vi "GitCheckProcRepo.vi"(8 "error in (no error)":errorcluster, 9 "Directory":path=path "", 11 "Git exec":string="git") -> (0 "error out":errorcluster, 1 "Directory out":path, 2 "ProcedureRepo?":bool, 3 "Git exec out":string="git")   [LabVIEW 2013]
uses:
  GitInterface/GitCmd.vi
  <vilib>/dlg_ctls.llb/Space Constant.vi
  PathtoDirPath.vi
  <vilib>/Platform/system.llb/System Exec.vi
  <vilib>/Utility/error.llb/Error Cluster From Error Code.vi
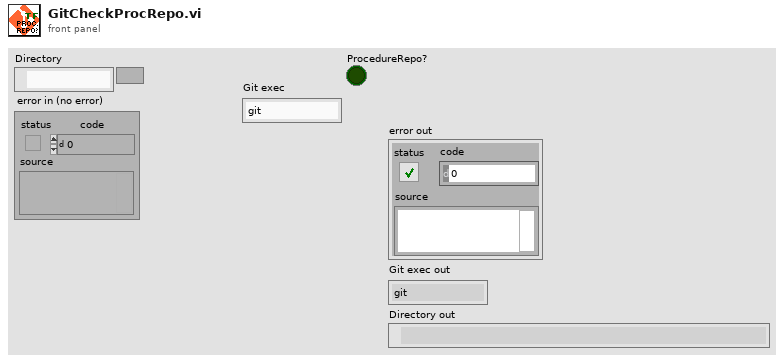
[diagram p1: front panel]
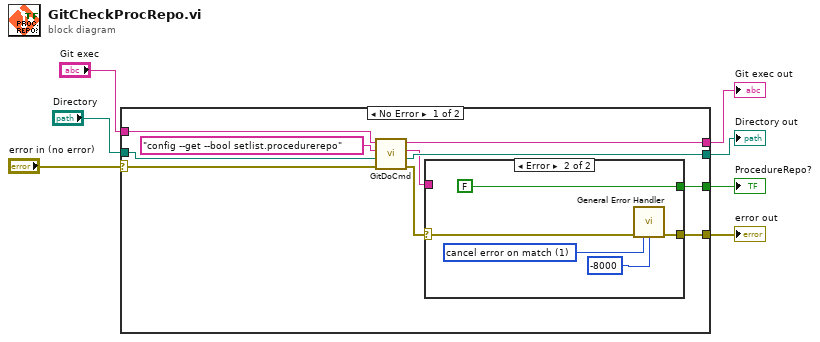
[diagram p0: block diagram]
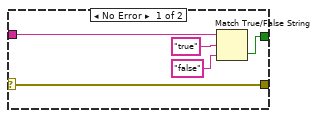
[diagram p2: hidden frame]
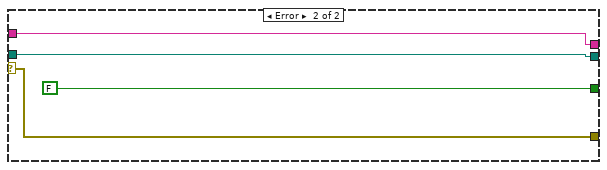
[diagram p3: hidden frame]
diagram:
  n1 = case shown="No Error" "error in (no error)" {
    selector: "error in (no error)" -> [w17 w31]
    tunnel: "Git exec" -> [w15 w29]
    tunnel: "Directory" -> [w16 w30]
    tunnel: [w12 FALSE ("selection")] -> w1
    tunnel: [w8 w31] -> w5
    tunnel: [w13 w30] -> w3
    tunnel: [w10 w29] -> w2
    frame No Error {
      n2 = call "GitDoCmd.vi"("error in (no error)"=w17, "Working Path"=w16, "Git command"="config --get --bool setlist.procedurerepo" ("string"), "Git exec"=w15) -> ("error out"=w9:errorcluster, "Working Path out"=w13:path, "Returned stdout"=w11:string, "Git exec out"=w10:string)  [unwired: 3 in]
      n3 = case shown="Error" w9 {
        selector: w9 -> [w18 w25]
        tunnel: [w20 FALSE ("selection")] -> w12
        tunnel: w11 -> [w19 _]
        tunnel: [w18 w24] -> w8
        frame No Error {
          n4 = Match True/False String(2:"false" ("false string"), 3:"true" ("true string"), 4:w19) -> (0:w20:bool)  [unwired: 1 out]
        }
        frame Error {
          w26 = 1 items=["no exception", "cancel error on match", "set error on match"] ("[exception action] (none:0)")
          n5 = call <vilib>:"General Error Handler.vi"("error in (no error)"=w25, "[exception action] (none:0)"=w26, "[exception code]"=-8000) -> ("error out"=w24:errorcluster)  [unwired: 8 in, 4 out]
        }
      }
    }
    frame Error {
    }
  }
  "error out" <- w5
  "Git exec out" <- w2
  "Directory out" <- w3
  "ProcedureRepo?" <- w1
